vi "Registers.Initialize.vi"(7 "Sample rate (Hz)":u32, 8 "error in (no error)":errorcluster, 9 "Values":dbl[](array[numeric]), 10 "Registers":T1[](array[typedef]) {"Register"."Data Type" format="%.0x"}, 11 "FPGA Ref":refnum<k20>) -> (0 "error out":errorcluster, 2 "Registers Ref":T4[](array[typedef]) {"Data Type" format="%.0x"}, 3 "FPGA Ref out":refnum<k20>)   [LabVIEW 2015, in "Fuel Injection Addon Engine.lvlib"]
uses:
  Fuel Injection Addon Engine.lvlib
  Types/FPGA Refs.ctl
  Shared/Types/FPGA Data Types.ctl
  Shared/Types/VS.Register.Info.ctl
  Shared/Types/Register.Info.ctl
  Shared/Fuel Injection Addon Shared.lvlib
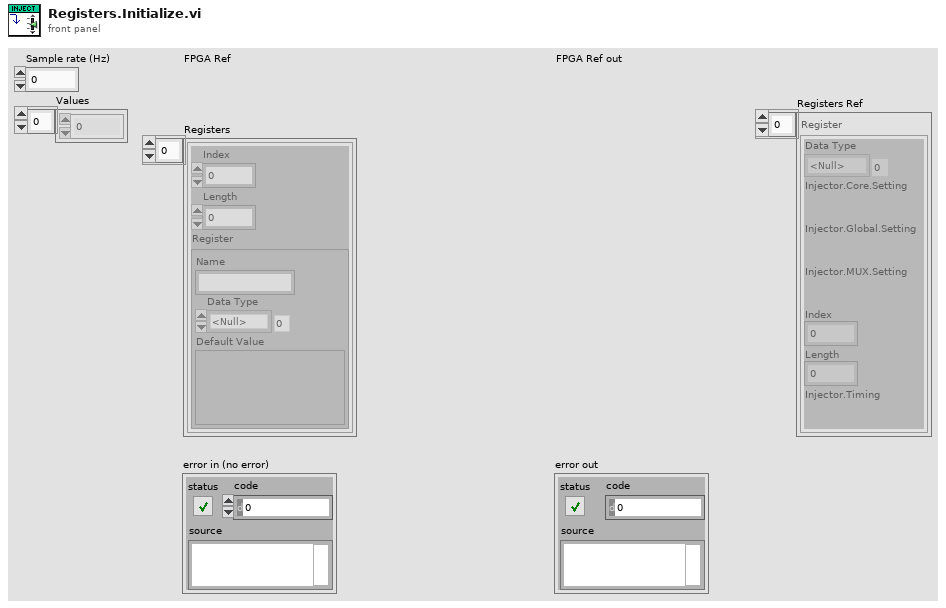
[diagram p1: front panel]
types:
  T1 = typedef "Fuel Injection Addon Shared.lvlib/VS.Register.Info.ctl" = cluster{"Index":i32, "Length":i32, "Register":T2}
  T2 = typedef "Fuel Injection Addon Shared.lvlib/Register.Info.ctl" = cluster{"Name":string, "Data Type":T3, "Default Value":variant}
  T3 = typedef "Fuel Injection Addon Shared.lvlib/FPGA Data Types.ctl" = enum8{"<Null>", "Injector.Core.Setting", "Injector.Global.Setting", "Injector.Mux.Setting", "Injector.Timing"}
  T4 = typedef "Fuel Injection Addon Engine.lvlib/FPGA Refs.ctl" = cluster{"Data Type":T3, "Injector.Core.Setting":refnum<k20>, "Injector.Global.Setting":refnum<k20>, "Injector.MUX.Setting":refnum<k20>, "Index":i32, "Length":i32, "Injector.Timing":refnum<k20>}
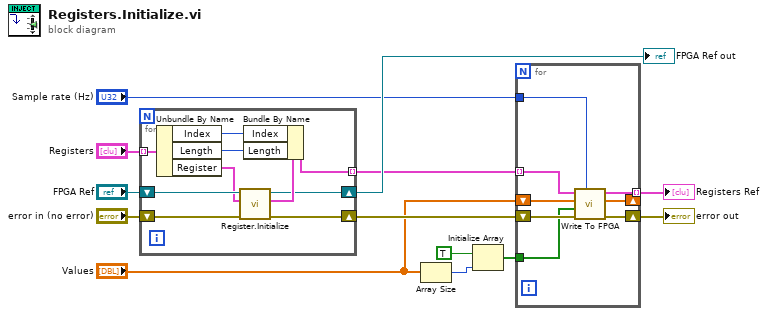
[diagram p0: block diagram]
diagram:
  n1 = for {
    shift-right: [w14] -> w5
    shift-left: "FPGA Ref" -> [w19]
    tunnel: [w23] -> w4 mode=indexing
    tunnel: "Registers" -> [w22] mode=indexing
    shift-right: [w15] -> w9
    shift-left: "error in (no error)" -> [w18]
    n2 = Unbundle By Name(w22) -> ("Index"=w20:i32, "Length"=w21:i32, "Register"=w16:T2)
    n3 = call "Register.Initialize.vi"("error in (no error)"=w18, "Register"=w16, "FPGA Ref"=w19) -> ("error out"=w15:errorcluster, "Register out"=w17:T4, "FPGA Ref out"=w14:refnum<k20>)  [unwired: 6 in]
    n4 = Bundle By Name(cluster=w17, "Index"=w20, "Length"=w21) -> (w23:T4)
  }
  "FPGA Ref out" <- w5
  n5 = Array Size(array="Values") -> (size(s)=w8:i32)
  n6 = Initialize Array(TRUE, w8) -> (w6:bool[])
  n7 = for {
    shift-right: [w27] -> _
    shift-left: "Values" -> [w28]
    shift-right: [w30] -> w10
    shift-left: w9 -> [w31]
    tunnel: w6 -> [w29]
    tunnel: "Sample rate (Hz)" -> [w26]
    tunnel: w4 -> [w25] mode=indexing
    tunnel: [w24] -> w3 mode=indexing
    n8 = call "Write To FPGA.vi"("Sample Rate"=w26, "error in (no error)"=w31, "Changed?"=w29, "Values"=w28, "FPGA Refs"=w25) -> ("error out"=w30:errorcluster, "Values out"=w27:dbl[], "FPGA Refs"=w24:T4)  [unwired: 4 in]
  }
  "error out" <- w10
  "Registers Ref" <- w3
